vi "Publish Pages.vi"(7 "Parallel?":bool, 8 "error in (no error)":errorcluster {"code" format="Error %.0f"}, 11 "VIDoc Printer - Confluence In":refnum<class "VIDoc Printer - Confluence.lvclass">) -> (0 "error out":errorcluster {"code" format="Error %.0f"}, 3 "VIDoc Printer - Confluence Out":refnum<class "VIDoc Printer - Confluence.lvclass">)   [LabVIEW 2023, in "VIDoc Printer - Confluence.lvlib" / "VIDoc Printer - Confluence.lvclass"]
uses:
  VIDoc Printer - Confluence.lvclass
  C:/projects/DMC/Tooling/Git-Action-Service/Source/Documentation Generation/Printers/Printer/VIDoc Printer.lvclass
  VIDoc Printer - Confluence.lvclass/VIDoc Printer - Confluence.ctl
  Printer/VIDoc Printer.lvclass
  UI Interaction/UI Interaction.lvclass
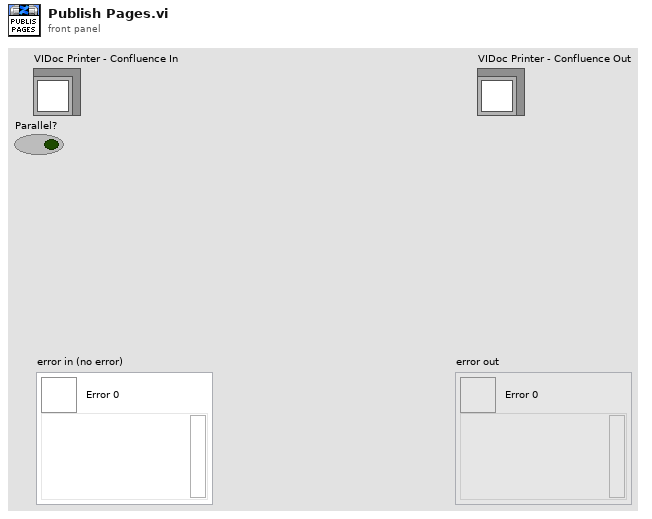
[diagram p1: front panel]
types:
  T1 = typedef "VIDoc Printer - Confluence.lvlib/VIDoc Printer - Confluence.lvclass/Page Info.ctl" = cluster{"Page":refnum<class "Page.lvclass">, "Content":string, "Attachments":set{path}}
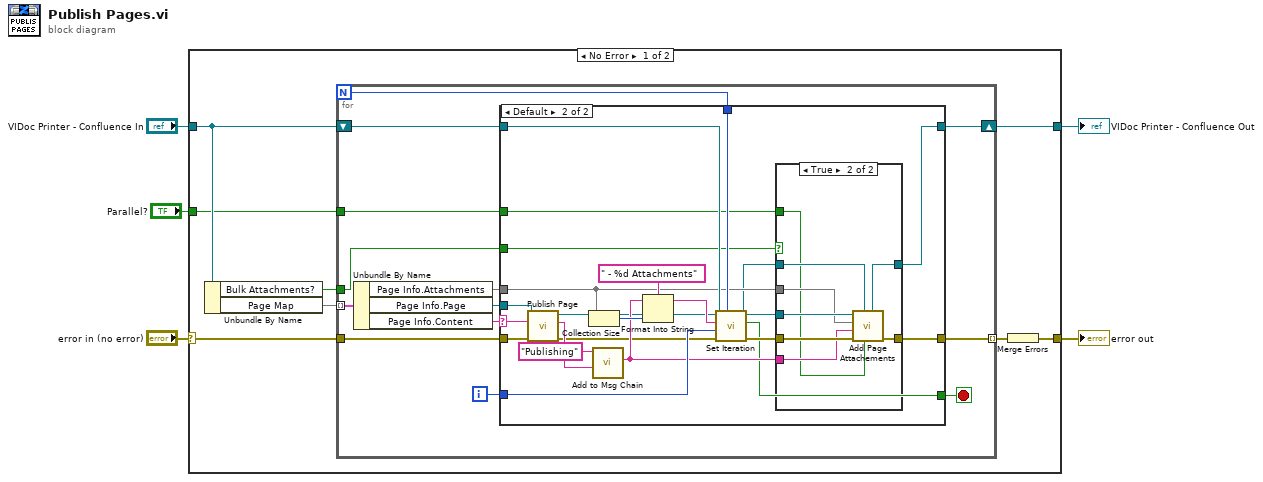
[diagram p0: block diagram]
diagram:
  n1 = case shown="No Error" "error in (no error)" {
    selector: "error in (no error)" -> [w11 w62]
    tunnel: [w7 w62] -> w4
    tunnel: [w10 w61] -> w2
    tunnel: "VIDoc Printer - Confluence In" -> [w9 w61]
    tunnel: "Parallel?" -> [w6 _]
    frame No Error {
      n2 = Unbundle By Name(w9) -> ("Bulk Attachments?"=w8:bool, "Page Map"=w12:map{string, T1})
      n3 = for {
        N -> [w23]
        tunnel: w12 -> [w26] mode=indexing
        shift-right: [w20] -> w10
        shift-left: w9 -> [w22]
        tunnel: w11 -> [w19]
        tunnel: [w16] -> w13 mode=indexing
        tunnel: w8 -> [w17]
        tunnel: w6 -> [w15]
        i -> [w24]
        stop <- w14 stop-if-true
        n4 = Unbundle By Name(w26) -> ("Page Info.Attachments"=w18:set{path}, "Page Info.Page"=w25:refnum<class "Page.lvclass">, "Page Info.Content"=w21:string)
        n5 = case shown="Default" w21 {
          selector: w21 -> [_ w32]
          tunnel: [w27 w45] -> w16
          tunnel: w25 -> [_ w33]
          tunnel: w24 -> [_ w50]
          tunnel: w23 -> [_ w49]
          tunnel: w22 -> [w28 w48]
          tunnel: [w28 w36] -> w20
          tunnel: w19 -> [w27 w34]
          tunnel: w18 -> [_ w40]
          tunnel: w17 -> [_ w39]
          tunnel: w15 -> [_ w38]
          tunnel: [_ w35] -> w14
          frame "" {
            # "Content was never added so don't attempt to edit the pages. \nThis prevents editing of any pages that weren't autogenerated but under the top level."
          }
          frame Default {
            n6 = call "Publish Page.vi"("error in (no error)"=w34, "Content"=w32, "Page in"=w33) -> ("error out"=w29:errorcluster, "Title"=w30:string, "Page out"=w31:refnum<class "Page.lvclass">)  [unwired: 5 in, 1 out]
            n7 = Collection Size(1:w40) -> (0:w43:i32)
            n8 = call "Add to Msg Chain.vi"("New"=w30, "Msg Chain in"="Publishing") -> ("Msg Chain out"=w41:string)  [unwired: 9 in]
            n9 = Format Into String(format string=" - %d Attachments", initial string=w41, w43) -> (resulting string=w42:string)  [unwired: 1 in, 1 out]
            n10 = call "Set Iteration.vi"("Progress Max"=w49, "error in (no error)"=w29, "Progress Value"=w50, "Message (No Message Update)"=w42, "VIDoc Printer In"=w48) -> ("error out"=w46:errorcluster, "Abort?"=w35:bool, "VIDoc Printer Out"=w37:refnum<class "VIDoc Printer - Confluence.lvclass">)  [unwired: 4 in]
            n11 = case shown="True" w39 {
              tunnel: w46 -> [w52 w60]
              tunnel: [w52 w53] -> w45
              tunnel: w31 -> [_ w57]
              tunnel: w41 -> [_ w55]
              tunnel: w40 -> [_ w56]
              tunnel: w38 -> [_ w54]
              tunnel: w37 -> [w51 w59]
              tunnel: [w51 w58] -> w36
              frame False {
              }
              frame True {
                n12 = call "Add Page Attachements.vi"("Parallel?"=w54, "Conf Printer in"=w59, "error in (no error)"=w60, "Msg Chain in"=w55, "Attachments"=w56, "Page in"=w57) -> ("error out"=w53:errorcluster, "Conf Printer out"=w58:refnum<class "VIDoc Printer - Confluence.lvclass">)  [unwired: 3 in, 1 out]
              }
            }
          }
        }
      }
      n13 = Merge Errors(w13) -> (w7:errorcluster)
    }
    frame Error {
    }
  }
  "error out" <- w4
  "VIDoc Printer - Confluence Out" <- w2
